vi "2_front_controls_1_variable.vi"() -> ()   [LabVIEW 2013]
panel:
  out "Boolean 2":bool
  in  "Boolean":bool
  out "Lampe 2":bool
  out "Lampe 1":bool
  in  "Control 2":dbl
  in  "Control 1":dbl
  in  "stop":bool
  in  "y":dbl
  in  "x":dbl
  out "x+y":dbl
  # "Eine Moeglichkeit zwei Kontrollelemente fuer ein und dieselbe Variable zu haben.\nz.B. Wenn in zwei Tabs auf die selbe Variable zugegriffen werden soll.\n(Rechtsklick -> Visible Items -> \"Digital Display\" loest dieses Problem nicht.)"
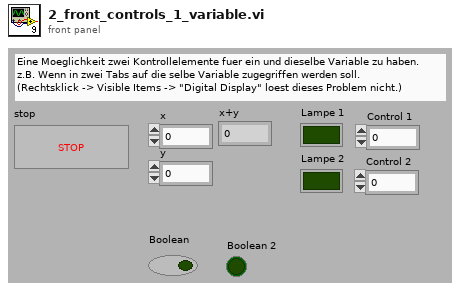
[diagram p1: front panel]
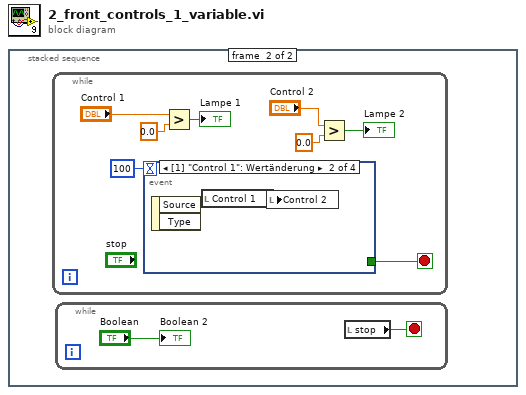
[diagram p0: block diagram]
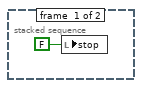
[diagram p2: hidden frame]
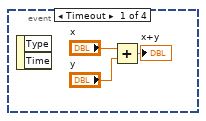
[diagram p3: hidden frame]
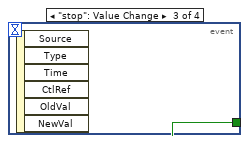
[diagram p4: hidden frame]
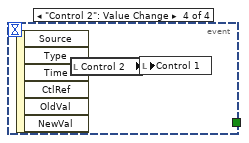
[diagram p5: hidden frame]
diagram:
  n1 = stacked-sequence {
    frame #0 {
      n2 = local write "stop"(FALSE ("stop")) -> ()
    }
    frame #1 {
      n3 = while {
        stop <- w5 stop-if-true
        n4 = event shown="[1] \"Control 1\": Wertänderung" {
          selector: _ -> [_ _ _ _]
          dyn-events: _ -> [_ _ _ _]
          timeout: 100 -> [_ _ _ _]
          tunnel: [_ _ TRUE _] -> w5
          event Timeout {
            n5 = event-data() -> ()  [unwired: 1 in, 2 out]
            n6 = Add(x="x", y="y") -> (x+y=→"x+y":dbl)
          }
          event "Control 1": Value Change {
            n7 = event-data() -> ()  [unwired: 1 in, 2 out]
            n8 = local read "Control 1"() -> (w15:dbl)
            n9 = local write "Control 2"(w15) -> ()
          }
          event "stop": Value Change {
            n10 = event-data() -> ()  [unwired: 1 in, 6 out]
          }
          event "Control 2": Value Change {
            n11 = event-data() -> ()  [unwired: 1 in, 6 out]
            n12 = local read "Control 2"() -> (w17:dbl)
            n13 = local write "Control 1"(w17) -> ()
          }
        }
        n14 = Greater?(x="Control 1", y=0.0) -> (0:→"Lampe 1":bool)
        n15 = Greater?(x="Control 2", y=0.0) -> (0:→"Lampe 2":bool)
      }
      n16 = while {
        stop <- w2 stop-if-true
        n17 = local read "stop"() -> (w2:bool)
        "Boolean 2" <- "Boolean"
      }
    }
  }
